vi "CreateProtectedEvents.vi"(8 "error in (no error)":errorcluster, 11 "SMO.UI.Splash":refnum<class "SMO.UI.Splash.lvclass">) -> (0 "error out":errorcluster, 3 "SMO.UI.Splash out":refnum<class "SMO.UI.Splash.lvclass">)   [LabVIEW 2013, in "SMO.UI.Splash.lvclass"]
doc: "JKI State Machine Objects (SMO) 1.0.0.5\nJKI - JKI\nCopyright (c) 2016, JKI"
uses:
  SMO.UI.Splash.lvclass
  <vilib>/JKI/JKI SMO/SMO.UI/SMO.UI.lvclass
  SMO.UI.Splash.lvclass/SMO.UI.Splash.ctl
panel:
  # "For instructions on how to use the JKI State Machine Objects, examples and video tutorials, visit:\nhttp://jki.net/state-machine-objects/\n\nJKI State Machine Objects™\nhttp://jki.net/state-machine-objects/\nCopyright (C) 2005-2015, JKI <info@jki.net>\nALL RIGHTS RESERVED"
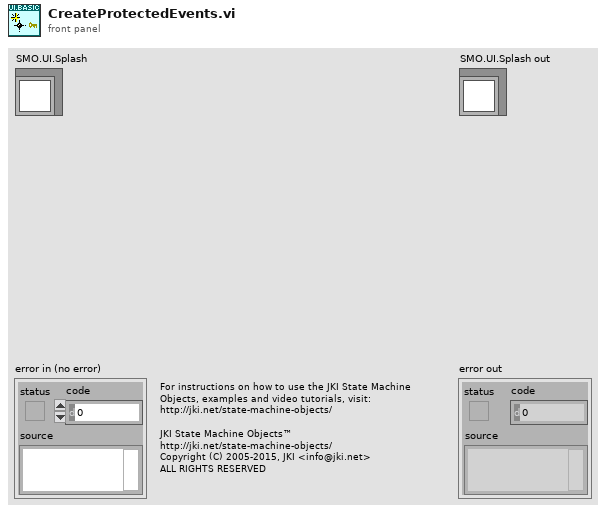
[diagram p1: front panel]
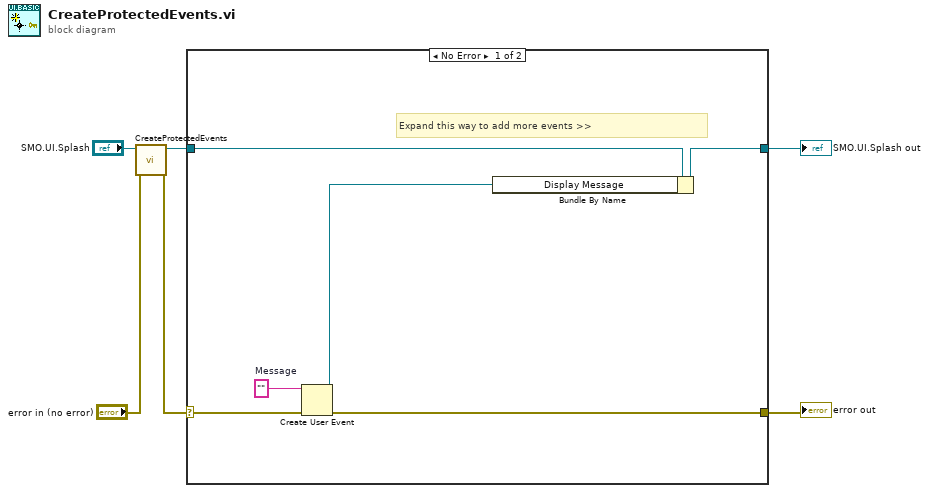
[diagram p0: block diagram]
diagram:
  n1 = call-parent "CreateProtectedEvents.vi"("error in (no error)"="error in (no error)", "SMO"="SMO.UI.Splash") -> ("error out"=w3:errorcluster, "SMO out"=w4:refnum<class "SMO.UI.Splash.lvclass">)  [unwired: 8 in]
  n2 = case shown="No Error" w3 {
    selector: w3 -> [w12 w14]
    tunnel: [w8 w14] -> w2
    tunnel: [w9 w13] -> w1
    tunnel: w4 -> [w10 w13]
    frame No Error {
      w7 = ""  # Message
      # "Expand this way to add more events >>"
      n3 = Create User Event(user event datatype=w7, error in=w12) -> (user event=w11:refnum<user-event>, error out=w8:errorcluster)
      n4 = Bundle By Name(cluster=w10, "Display Message"=w11) -> (w9:refnum<class "SMO.UI.Splash.lvclass">)
    }
    frame Error {
    }
  }
  "error out" <- w2
  "SMO.UI.Splash out" <- w1
